vi "Is Refnum.vi"(10 "Self":refnum<class "Msg Type Strategy.lvclass">) -> (2 "Error":errorcluster)   [LabVIEW 2021, in "jettl.lvlib" / "Error.lvlib"]
uses:
  Error.lvlib
  Msg Type Strategy/Msg Type Strategy/Msg Type Strategy.lvclass
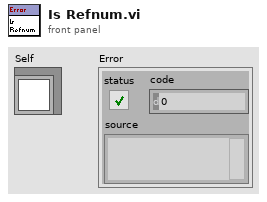
[diagram p1: front panel]
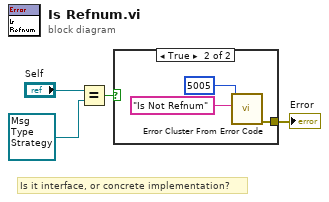
[diagram p0: block diagram]
diagram:
  # "Is it interface, or concrete implementation?"
  n1 = Equal?(x="Self", y=refnum<class "Msg Type Strategy.lvclass"> refnum) -> (x = y?=w1:bool)
  n2 = case shown="True" w1 {
    tunnel: [_ w7] -> w4
    frame False {
    }
    frame True {
      n3 = call <vilib>:"Error Cluster From Error Code.vi"("error message (\"\")"="Is Not Refnum" ("error message (\"\")"), "error code (0)"=5005) -> ("error out"=w7:errorcluster)  [unwired: 7 in]
    }
  }
  "Error" <- w4
